vi "pi_piezo_load_xml.vi"(8 "error in":errorcluster, 10 "child node in":refnum<k20>, 11 "PI_Piezo (in)":refnum<class "PI_Piezo.lvclass">) -> (0 "error out":errorcluster, 2 "child node out":refnum<k20>, 3 "PI_Piezo":refnum<class "PI_Piezo.lvclass">)   [LabVIEW 2013, in "PI_Piezo.lvclass"]
doc: "Loads analog output settings from xml. Expected format:\n\n<Enable>%b</Enable>\n<PhysicalChannel>%s</PhysicalChannel>\n<MinimumValue>%f</MinimumValue>\n<MaximumValue>%f</MaximumValue>\n<SamplesPerSecond>%f</SamplesPerSecond>\n<TotalAOTime units=\"seconds\">%s</TotalAOTime>\n<AnalogOutputEquations>\n%s</AnalogOutputEquations>\n<StartTrigger.WaitForStartTrigger>%b</StartTrigger.WaitForStartTrigger\n<StartTrigger.source>%s</StartTrigger.source>\n<StartTrigger.edge>%s</StartTrigger.edge>\n\nMTL 2012 Dec 31"
uses:
  PI_Piezo.lvclass
  PI_Piezo.lvclass/PI_Piezo.ctl
  piezo_controller.ctl
  piezo_channel.ctl
  <vilib>/xml/Close Reference(Node).vi
  <resource>/objmgr/DOMUserDefRef.rc
  <vilib>/xml/NI_XML.lvlib
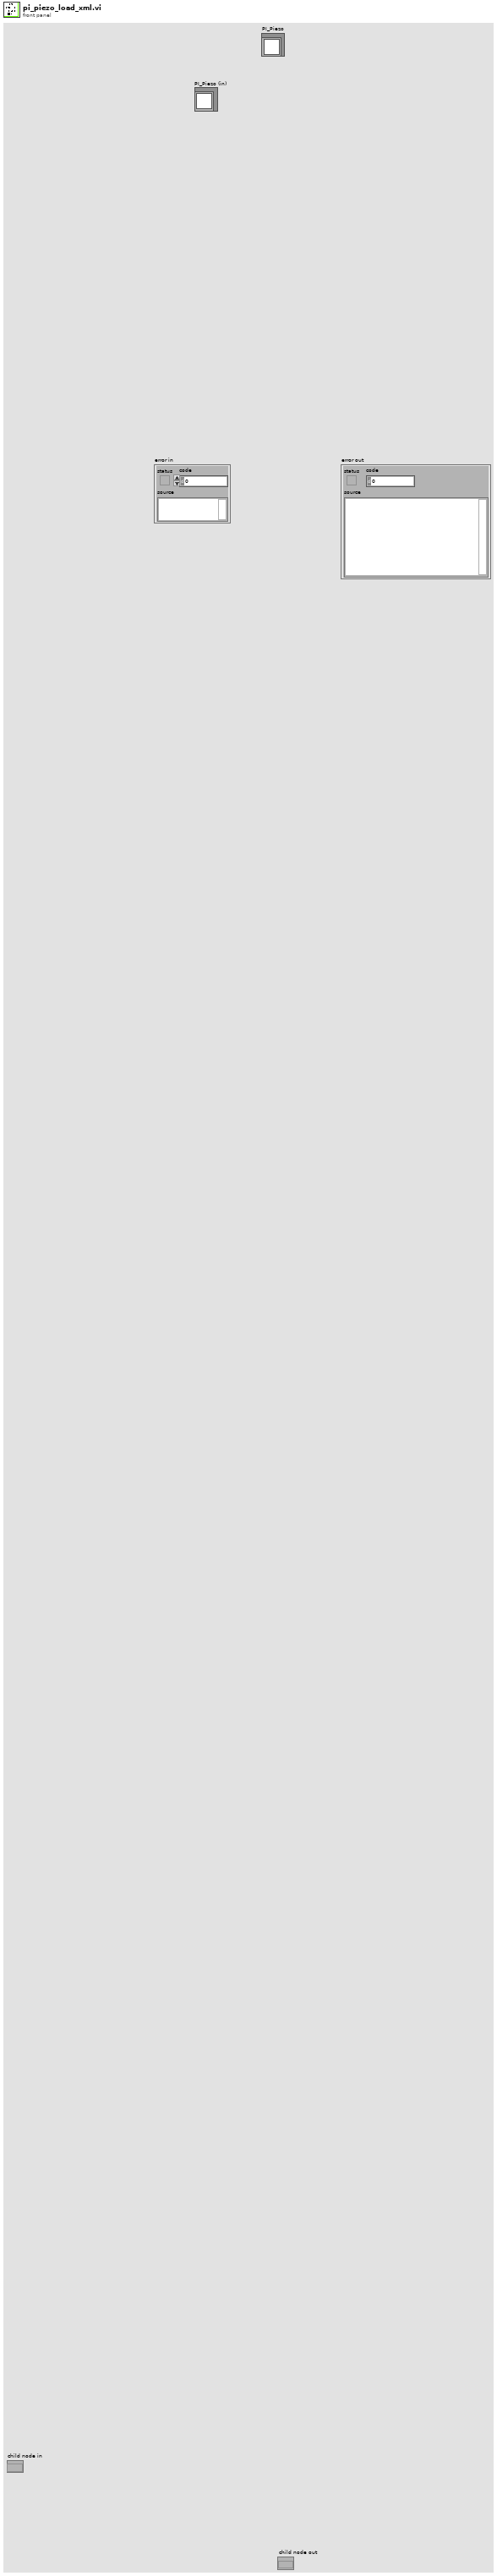
[diagram p1: front panel]
types:
  T1 = typedef "PI_Piezo.lvclass/piezo_channel.ctl" = cluster{"Servo":bool, "Set Position":dbl}
  T2 = typedef "PI_Piezo.lvclass/settings.ctl" = cluster{"Enable":bool, "Array of Piezo Controllers":T3[]}
  T3 = typedef "PI_Piezo.lvclass/piezo_controller.ctl" = cluster{"Enable":bool, "Serial No.":string, "Array of Piezo Channels":T1[]}
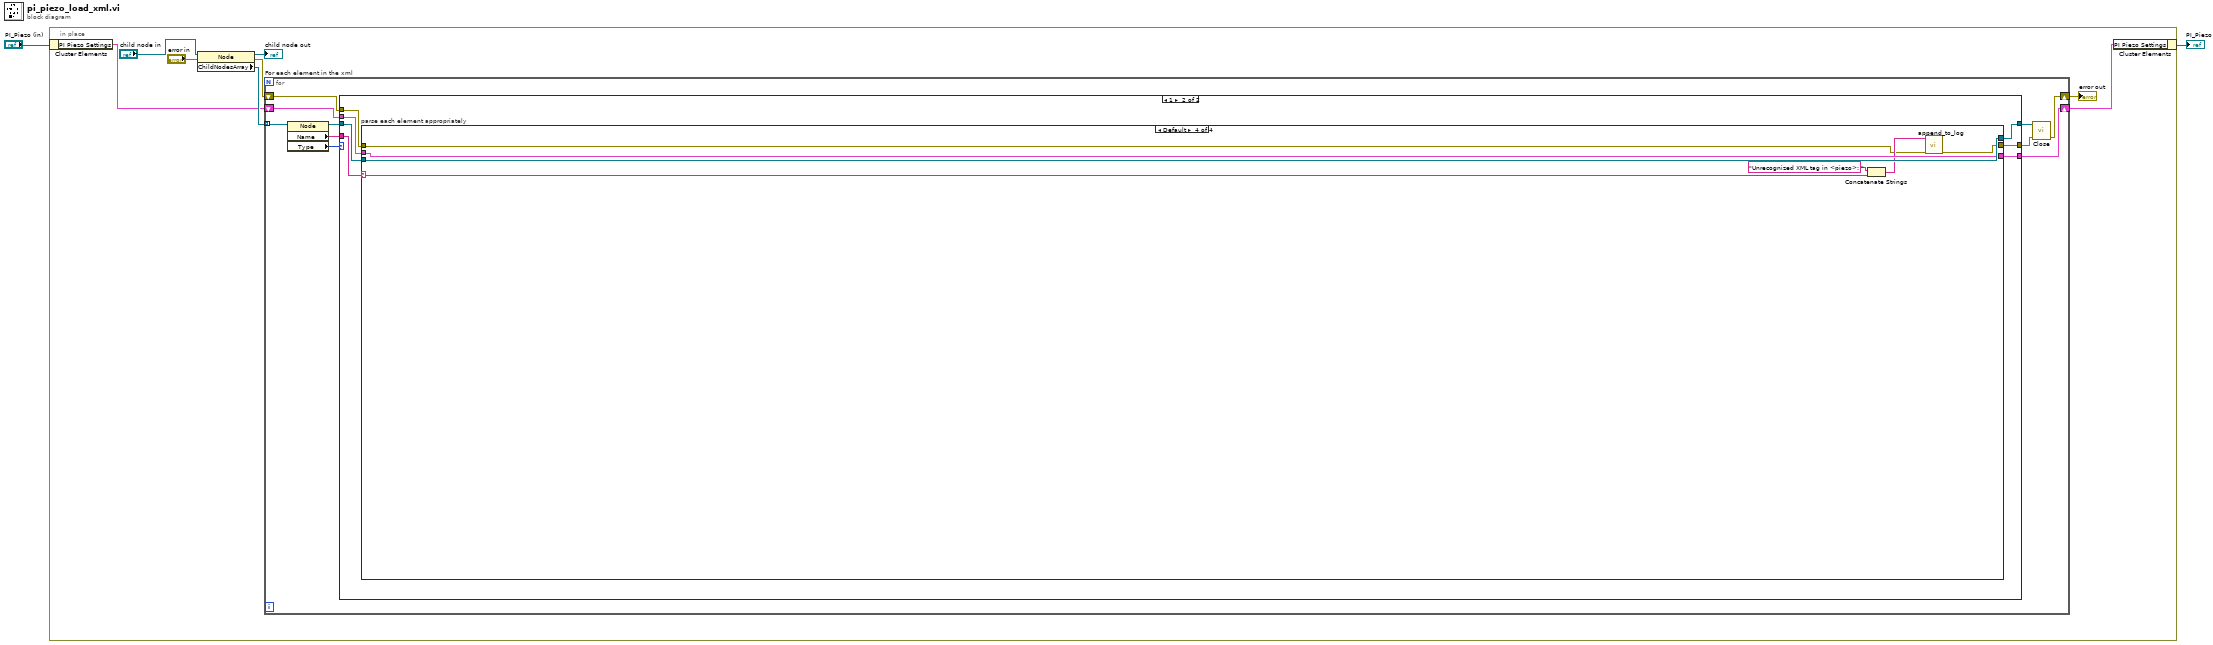
[diagram p0: block diagram]
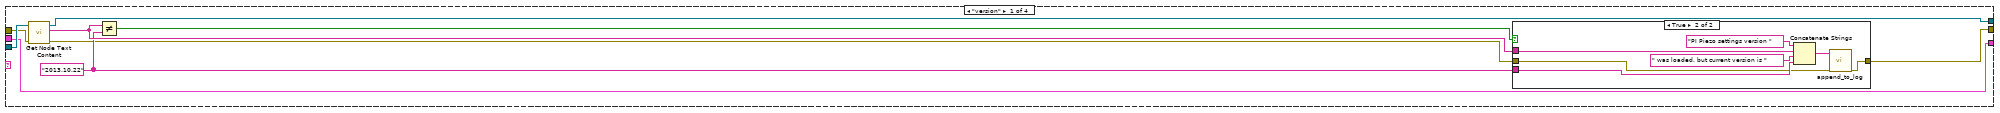
[diagram p3: hidden frame]
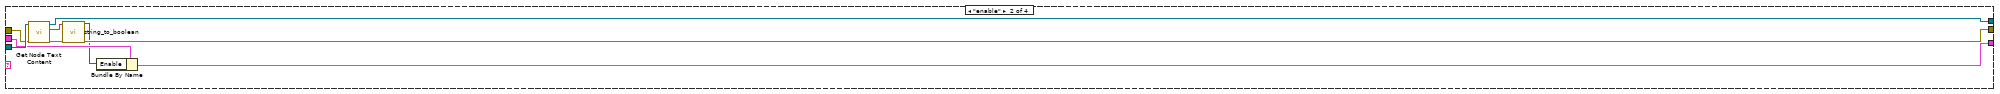
[diagram p5: hidden frame]
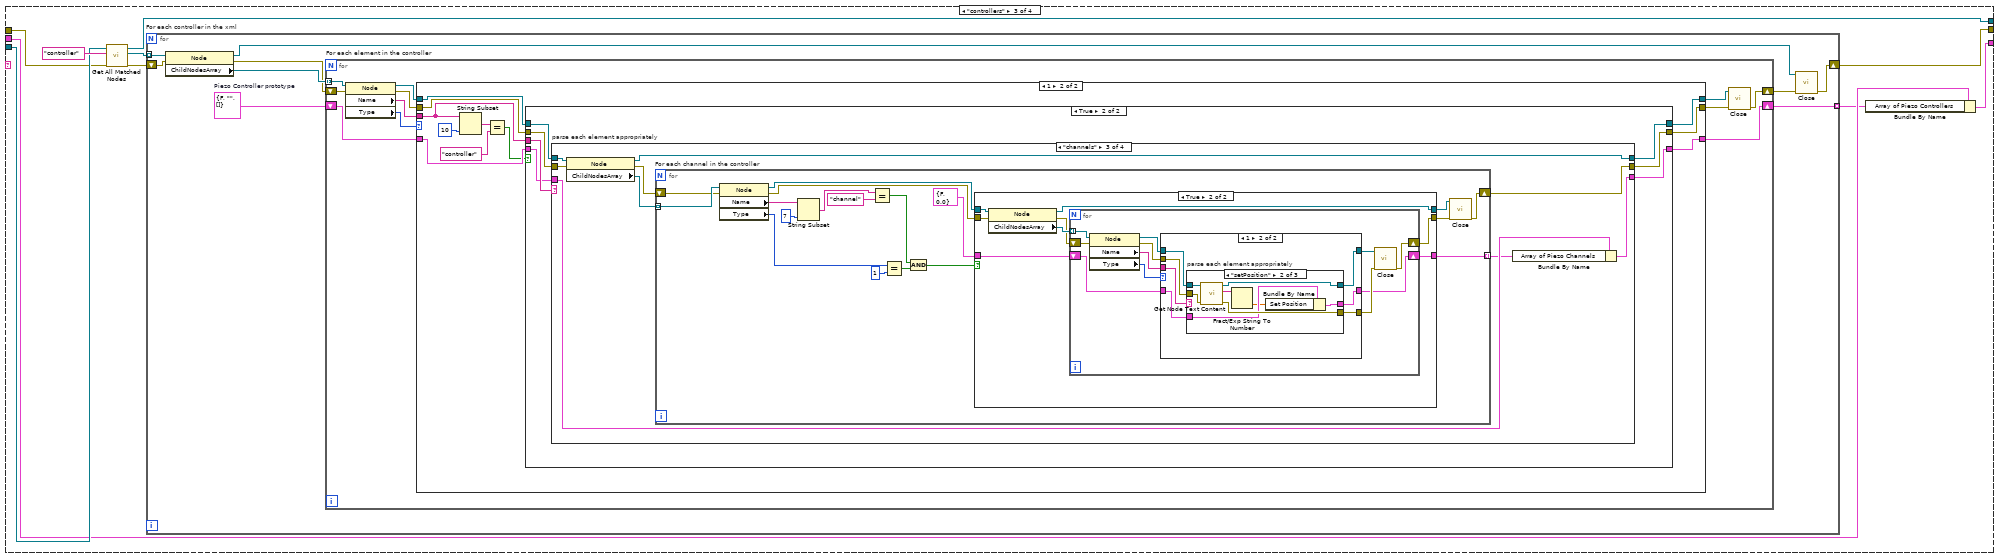
[diagram p6: hidden frame]
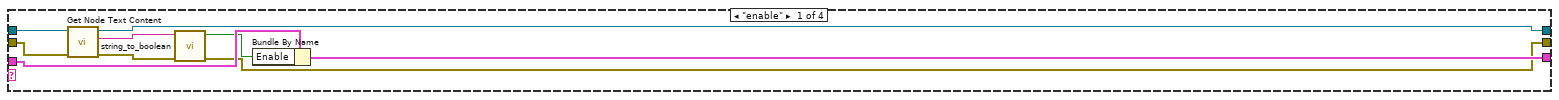
[diagram p9: hidden frame]
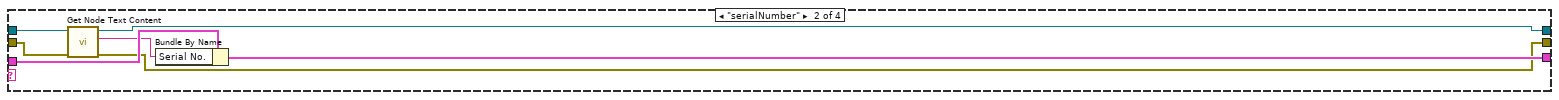
[diagram p10: hidden frame]
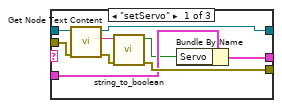
[diagram p13: hidden frame]
diagram:
  n1 = in-place {
    n2 = in-place-cluster #1("PI_Piezo (in)") -> ("PI Piezo Settings"=w4:T2)
    n3 = property class="Node"(reference="child node in", error in="error in") -> (reference out=→"child node out":refnum<k20>, error out=w6:errorcluster, "ChildNodesArray"=w7:refnum<k20>[])
    n4 = for "For each element in the xml" {
      tunnel: w7 -> [w20] mode=indexing
      shift-right: [w14] -> w5
      shift-left: w6 -> [w17]
      shift-right: [w12] -> w3
      shift-left: w4 -> [w13]
      n5 = property class="Node"(reference=w20) -> (reference out=w19:refnum<k20>, "Name"=w18:string, "Type"=w11:i32)  [unwired: 1 in, 1 out]
      n6 = case shown="1" w11 {
        tunnel: w19 -> [w23 w30]
        tunnel: w18 -> [_ w29]
        tunnel: w17 -> [w22 w28]
        tunnel: [w23 w27] -> w16
        tunnel: [w22 w26] -> w15
        tunnel: w13 -> [w21 w25]
        tunnel: [w21 w24] -> w12
        frame Default {
        }
        frame 1 {
          n7 = case "parse each element appropriately" shown="Default" w29 {
            selector: w29 -> [_ _ _ w209]
            tunnel: [w32 w50 w63 w215] -> w27
            tunnel: w30 -> [w35 w56 w62 w215]
            tunnel: w28 -> [w34 w55 w60 w211]
            tunnel: [w33 w49 w61 w210] -> w26
            tunnel: w25 -> [w31 w52 w58 w214]
            tunnel: [w31 w51 w59 w214] -> w24
            frame "version" {
              w37 = "2013.10.22" ("y")
              n8 = call <vilib>:"Get Node Text Content.vi"("error in (no error)"=w34, "node in"=w35) -> ("error out"=w36:errorcluster, "node text"=w38:string, "node out"=w32:refnum<k20>)  [unwired: 7 in]
              n9 = Not Equal?(x=w38, y=w37) -> (x != y?=w39:bool)
              n10 = case shown="True" w39 {
                tunnel: w38 -> [_ w46]
                tunnel: w37 -> [_ w44]
                tunnel: w36 -> [w40 w42]
                tunnel: [w40 w41] -> w33
                frame False {
                }
                frame True {
                  n11 = Concatenate Strings("PI Piezo settings version " ("string"), w46, " was loaded, but current version is " ("string"), w44) -> (w43:string)
                  n12 = call "append_to_log.vi"("error in"=w42, "string"=w43) -> ("error out"=w41:errorcluster)  [unwired: 9 in]
                }
              }
            }
            frame "enable" {
              n13 = call <vilib>:"Get Node Text Content.vi"("error in (no error)"=w55, "node in"=w56) -> ("error out"=w53:errorcluster, "node text"=w54:string, "node out"=w50:refnum<k20>)  [unwired: 7 in]
              n14 = call "string_to_boolean.vi"("error in"=w53, "string"=w54) -> ("error out"=w49:errorcluster, "boolean"=w48:bool)  [unwired: 8 in]
              n15 = Bundle By Name(cluster=w52, "Enable"=w48) -> (w51:T2)
            }
            frame "controllers" {
              n16 = call <vilib>:"Get All Matched Nodes.vi"("error in (no error)"=w60, "XPath expression"="controller", "node in"=w62) -> ("error out"=w65:errorcluster, "node result array"=w64:refnum<k20>[], "node out"=w63:refnum<k20>)  [unwired: 6 in]
              n17 = for "For each controller in the xml" {
                tunnel: w64 -> [w75] mode=indexing
                shift-right: [w69] -> w61
                shift-left: w65 -> [w74]
                tunnel: [w68] -> w57 mode=indexing
                w67 = T3 {"Enable"=FALSE, "Serial No."="", "Array of Piezo Channels"=[]}  # Piezo Controller prototype
                n18 = property class="Node"(reference=w75, error in=w74) -> (reference out=w71:refnum<k20>, error out=w72:errorcluster, "ChildNodesArray"=w73:refnum<k20>[])
                n19 = for "For each element in the controller" {
                  shift-right: [w79] -> w70
                  shift-left: w72 -> [w83]
                  tunnel: w73 -> [w86] mode=indexing
                  shift-right: [w77] -> w68
                  shift-left: w67 -> [w78]
                  n20 = property class="Node"(reference=w86, error in=w83) -> (reference out=w81:refnum<k20>, error out=w84:errorcluster, "Name"=w85:string, "Type"=w76:i32)
                  n21 = case shown="1" w76 {
                    tunnel: w85 -> [_ w95]
                    tunnel: w84 -> [w88 w100]
                    tunnel: [w89 w90] -> w82
                    tunnel: w81 -> [w89 w99]
                    tunnel: [w88 w98] -> w80
                    tunnel: w78 -> [w87 w97]
                    tunnel: [w87 w96] -> w77
                    frame Default {
                    }
                    frame 1 {
                      n22 = String Subset(string=w95, length (rest)=10 ("length (rest)")) -> (substring=w93:string)  [unwired: 1 in]
                      n23 = Equal?(x=w93, y="controller") -> (x = y?=w91:bool)
                      n24 = case shown="True" w91 {
                        tunnel: w95 -> [_ w110]
                        tunnel: w100 -> [w102 w109]
                        tunnel: w99 -> [w103 w107]
                        tunnel: [w102 w106] -> w98
                        tunnel: w97 -> [w101 w105]
                        tunnel: [w101 w104] -> w96
                        tunnel: [w103 w108] -> w90
                        frame False {
                        }
                        frame True {
                          n25 = case "parse each element appropriately" shown="\"channels\"" w110 {
                            tunnel: w109 -> [w118 w125 w129 w208]
                            tunnel: [w111 w120 w135 w208] -> w106
                            tunnel: [w115 w121 w127 w207] -> w108
                            tunnel: w107 -> [w119 w126 w131 w207]
                            tunnel: w105 -> [w117 w124 w133 w206]
                            tunnel: [w116 w123 w134 w206] -> w104
                            frame "enable" {
                              n26 = call <vilib>:"Get Node Text Content.vi"("error in (no error)"=w118, "node in"=w119) -> ("error out"=w112:errorcluster, "node text"=w114:string, "node out"=w115:refnum<k20>)  [unwired: 7 in]
                              n27 = call "string_to_boolean.vi"("error in"=w112, "string"=w114) -> ("error out"=w111:errorcluster, "boolean"=w113:bool)  [unwired: 8 in]
                              n28 = Bundle By Name(cluster=w117, "Enable"=w113) -> (w116:T3)
                            }
                            frame "serialNumber" {
                              n29 = call <vilib>:"Get Node Text Content.vi"("error in (no error)"=w125, "node in"=w126) -> ("error out"=w120:errorcluster, "node text"=w122:string, "node out"=w121:refnum<k20>)  [unwired: 7 in]
                              n30 = Bundle By Name(cluster=w124, "Serial No."=w122) -> (w123:T3)
                            }
                            frame "channels" {
                              n31 = property class="Node"(reference=w131, error in=w129) -> (reference out=w127:refnum<k20>, error out=w128:errorcluster, "ChildNodesArray"=w130:refnum<k20>[])
                              n32 = for "For each channel in the controller" {
                                shift-right: [w153] -> w135
                                shift-left: w128 -> [w148]
                                tunnel: w130 -> [w149] mode=indexing
                                tunnel: [w151] -> w132 mode=indexing
                                n33 = property class="Node"(reference=w149, error in=w148) -> (reference out=w147:refnum<k20>, error out=w137:errorcluster, "Name"=w146:string, "Type"=w140:i32)
                                n34 = String Subset(string=w146, length (rest)=7 ("length (rest)")) -> (substring=w144:string)  [unwired: 1 in]
                                n35 = Equal?(x=w144, y="channel" ("XPath expression")) -> (x = y?=w141:bool)
                                n36 = Equal?(x=w140, y=1) -> (x = y?=w138:bool)
                                n37 = And(x=w141, y=w138) -> (x .and. y?=w142:bool)
                                n38 = case shown="True" w142 {
                                tunnel: w147 -> [w155 w164]
                                tunnel: w137 -> [w156 w163]
                                tunnel: [w155 w162] -> w152
                                tunnel: [w154 w159] -> w151
                                tunnel: [w156 w158] -> w150
                                tunnel: T1 {"Servo"=FALSE, "Set Position"=0.0} ("Piezo Channel") -> [w154 w157]
                                frame False {
                                }
                                frame True {
                                n39 = property class="Node"(reference=w164, error in=w163) -> (reference out=w162:refnum<k20>, error out=w160:errorcluster, "ChildNodesArray"=w161:refnum<k20>[])
                                n40 = for {
                                tunnel: w161 -> [w175] mode=indexing
                                shift-right: [w169] -> w158
                                shift-left: w160 -> [w173]
                                shift-right: [w166] -> w159
                                shift-left: w157 -> [w167]
                                n41 = property class="Node"(reference=w175, error in=w173) -> (reference out=w171:refnum<k20>, error out=w172:errorcluster, "Name"=w174:string, "Type"=w165:i32)
                                n42 = case shown="1" w165 {
                                tunnel: w174 -> [_ w185]
                                tunnel: w172 -> [w177 w184]
                                tunnel: w171 -> [w178 w183]
                                tunnel: [w178 w182] -> w170
                                tunnel: [w177 w181] -> w168
                                tunnel: w167 -> [w176 w180]
                                tunnel: [w176 w179] -> w166
                                frame Default {
                                }
                                frame 1 {
                                n43 = case "parse each element appropriately" shown="\"setPosition\"" w185 {
                                tunnel: [w189 w202 w205] -> w181
                                tunnel: [w194 w201 w203] -> w182
                                tunnel: [w193 w200 w204] -> w179
                                tunnel: w184 -> [w192 w198 w205]
                                tunnel: w183 -> [w191 w199 w203]
                                tunnel: w180 -> [w188 w197 w204]
                                frame "setServo" {
                                n44 = call <vilib>:"Get Node Text Content.vi"("error in (no error)"=w192, "node in"=w191) -> ("error out"=w190:errorcluster, "node text"=w186:string, "node out"=w194:refnum<k20>)  [unwired: 7 in]
                                n45 = call "string_to_boolean.vi"("error in"=w190, "string"=w186) -> ("error out"=w189:errorcluster, "boolean"=w187:bool)  [unwired: 8 in]
                                n46 = Bundle By Name(cluster=w188, "Servo"=w187) -> (w193:T1)
                                }
                                frame "setPosition" {
                                n47 = call <vilib>:"Get Node Text Content.vi"("error in (no error)"=w198, "node in"=w199) -> ("error out"=w202:errorcluster, "node text"=w196:string, "node out"=w201:refnum<k20>)  [unwired: 7 in]
                                n48 = Fract/Exp String To Number(string=w196) -> (number=w195:dbl)  [unwired: 3 in, 1 out]
                                n49 = Bundle By Name(cluster=w197, "Set Position"=w195) -> (w200:T1)
                                }
                                frame Default {
                                }
                                }
                                }
                                }
                                n50 = call-poly <vilib>:"Close.vi"("error in (no error)"=w168, "node"=w170) -> ("error out"=w169:errorcluster)  [unwired: 7 in]
                                }
                                }
                                }
                                n51 = call-poly <vilib>:"Close.vi"("error in (no error)"=w150, "node"=w152) -> ("error out"=w153:errorcluster)  [unwired: 7 in]
                              }
                              n52 = Bundle By Name(cluster=w133, "Array of Piezo Channels"=w132) -> (w134:T3)
                            }
                            frame "None", Default {
                            }
                          }
                        }
                      }
                    }
                  }
                  n53 = call-poly <vilib>:"Close.vi"("error in (no error)"=w80, "node"=w82) -> ("error out"=w79:errorcluster)  [unwired: 7 in]
                }
                n54 = call-poly <vilib>:"Close.vi"("error in (no error)"=w70, "node"=w71) -> ("error out"=w69:errorcluster)  [unwired: 7 in]
              }
              n55 = Bundle By Name(cluster=w58, "Array of Piezo Controllers"=w57) -> (w59:T2)
            }
            frame Default {
              n56 = Concatenate Strings("Unrecognized XML tag in <piezo>: " ("string"), w209) -> (w212:string)
              n57 = call "append_to_log.vi"("error in"=w211, "string"=w212) -> ("error out"=w210:errorcluster)  [unwired: 9 in]
            }
          }
        }
      }
      n58 = call-poly <vilib>:"Close.vi"("error in (no error)"=w15, "node"=w16) -> ("error out"=w14:errorcluster)  [unwired: 7 in]
    }
    "error out" <- w5
    n59 = in-place-cluster #1("PI Piezo Settings"=w3) -> (→"PI_Piezo":refnum<class "PI_Piezo.lvclass">)
  }
